vi "CalculateBestY.vi"(8 "error in (no error)":errorcluster, 9 "Point":dbl[](array[numeric]), 10 "Game":refnum<class "Game.lvclass">, 11 "SupportAttackerPosition in":refnum<class "SupportAttackerPosition.lvclass">) -> (0 "error out":errorcluster, 2 "reference out":refnum<class "Game.lvclass">, 3 "SupportAttackerPosition out":refnum<class "SupportAttackerPosition.lvclass">)   [LabVIEW 2023, in "SupportAttackerPosition.lvclass"]
uses:
  SupportAttackerPosition.lvclass
  Game_class/Game.lvclass
  Game_class/Game.lvclass/Game.ctl
  Game_class/Read Utilities.lvclass.vi
  Game_class/Write Utilities.lvclass.vi
  Utilities_class/Utilities.lvclass
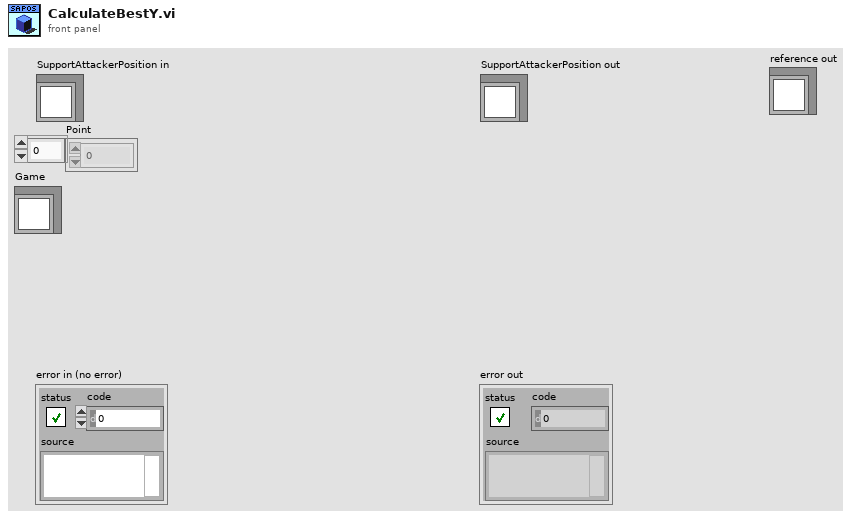
[diagram p1: front panel]
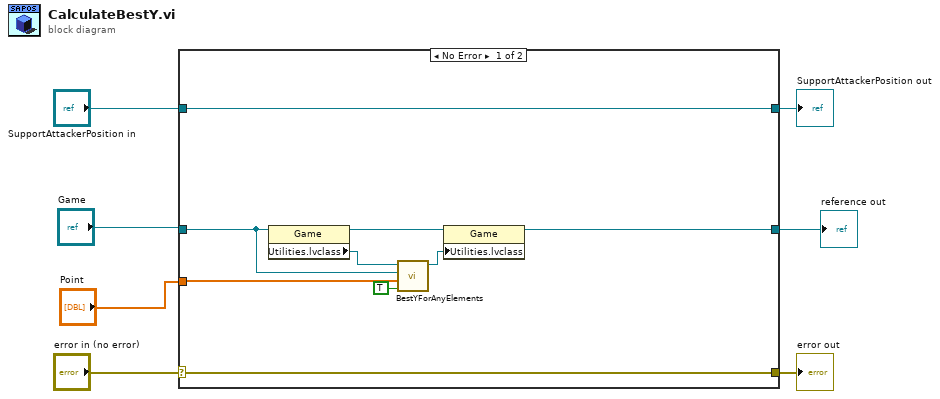
[diagram p0: block diagram]
diagram:
  n1 = case shown="No Error" "error in (no error)" {
    selector: "error in (no error)" -> [w15 w19]
    tunnel: [w15 w19] -> w6
    tunnel: [w16 w18] -> w4
    tunnel: "SupportAttackerPosition in" -> [w16 w18]
    tunnel: "Game" -> [w10 w17]
    tunnel: "Point" -> [w9 _]
    tunnel: [w8 w17] -> w1
    frame No Error {
      n2 = property class="Game"(reference=w10) -> (reference out=w11:refnum<class "Game.lvclass">, "Utilities.lvclass"=w14:refnum<class "Utilities.lvclass">)  [unwired: 1 in, 1 out]
      n3 = call "BestYForAnyElements.vi"("inimigos"=TRUE, "Position to be analyzed"=w9, "Game"=w10, "Utilities in"=w14) -> ("Utilities out"=w12:refnum<class "Utilities.lvclass">)  [unwired: 4 in, 3 out]
      n4 = property class="Game"(reference=w11, "Utilities.lvclass"=w12) -> (reference out=w8:refnum<class "Game.lvclass">)  [unwired: 1 in, 1 out]
    }
    frame Error {
    }
  }
  "error out" <- w6
  "SupportAttackerPosition out" <- w4
  "reference out" <- w1
